vi "Do.vi"(8 "error in (no error)":errorcluster, 10 "Actor in":refnum<class "Actor.lvclass">, 11 "Multiplication Result Msg":refnum<class "Multiplication Result Msg.lvclass">) -> (0 "error out":errorcluster, 2 "Actor out":refnum<class "Actor.lvclass">)   [LabVIEW 2024, in "Multiplication Result Msg.lvclass"]
doc: "(<B>Filename</B>: Actor Framework.lvlib:Message.lvclass:Do.vi)\n\nDefines what a message does when it is received by an actor. Generally, a message instructs an actor to invoke one of its methods. By default, this method does nothing. A child class must override it to define behavior. Create a child class by using the Actor Framework Message Maker dialog box."
uses:
  Multiplication Result Msg.lvclass
  <vilib>/ActorFramework/Actor/Actor.lvclass
  Calculator Actor Class/Calculator Actor.lvclass
  C:/Program Files/National Instruments/LabVIEW 2024/vi.lib/ActorFramework/Actor/Actor.lvclass
  Multiplication Result Msg.lvclass/Multiplication Result Msg.ctl
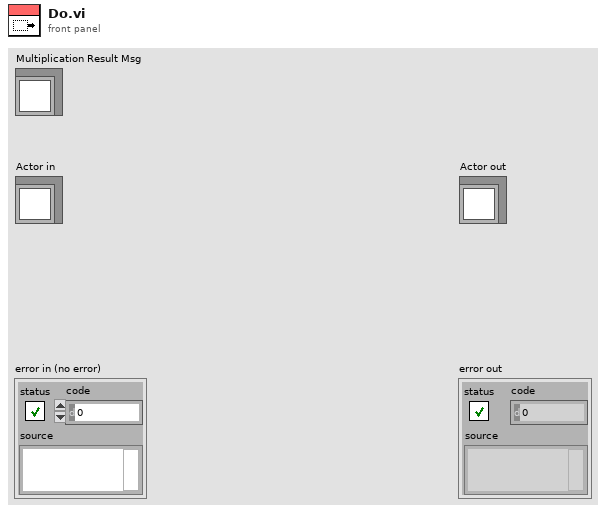
[diagram p1: front panel]
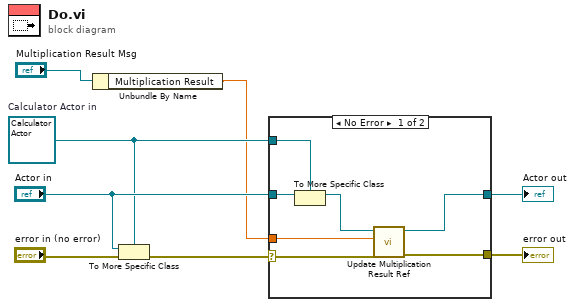
[diagram p0: block diagram]
diagram:
  w4 = refnum<class "Calculator Actor.lvclass"> refnum  # Calculator Actor in
  n1 = Unbundle By Name("Multiplication Result Msg") -> ("Multiplication Result"=w1:dbl)
  n2 = To More Specific Class(target class=w4, reference="Actor in", error in="error in (no error)") -> (error out=w6:errorcluster)  [unwired: 1 out]
  n3 = case shown="No Error" w6 {
    selector: w6 -> [w14 w16]
    tunnel: "Actor in" -> [w15 w17]
    tunnel: [w13 w16] -> w5
    tunnel: w4 -> [w12 _]
    tunnel: [w10 w17] -> w3
    tunnel: w1 -> [w9 _]
    frame No Error {
      n4 = To More Specific Class(target class=w12, reference=w15) -> (specific class reference=w11:refnum<class "Calculator Actor.lvclass">)  [unwired: 1 in, 1 out]
      n5 = call "Update Multiplication Result Ref.vi"("error in (no error)"=w14, "Multiplication Result"=w9, "Calculator Actor in"=w11) -> ("error out"=w13:errorcluster, "Calculator Actor out"=w10:refnum<class "Calculator Actor.lvclass">)  [unwired: 7 in]
    }
    frame Error {
    }
  }
  "error out" <- w5
  "Actor out" <- w3
